vi "SRV_Write_Comm.vi"(8 "error in (no error)":errorcluster, 10 "Command Sent":string, 11 "SRV In":refnum<k5>) -> (0 "error out":errorcluster, 2 "Command Sent dup":string, 3 "SRV Out":refnum<k5>)   [LabVIEW 2014]
doc: "Writes a string to the SRV.\n\n\nWritten for Benilde St. Margaret's School - Tim Jump\nBy Doug Schmertman - Logic PD\nCopyright 2012"
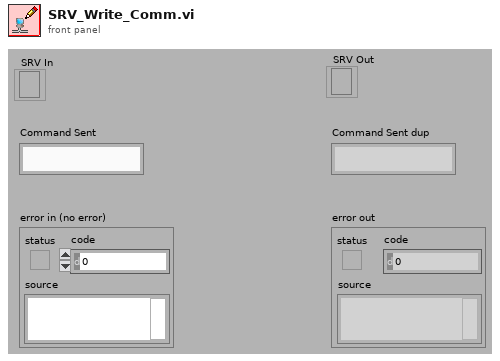
[diagram p1: front panel]
types:
  T1 = typedef "SRV_PM_Packet Mode Style.ctl" = enum16{"Old", "New PM"}
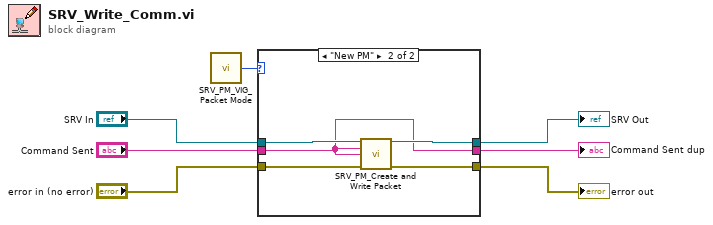
[diagram p0: block diagram]
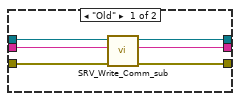
[diagram p2: hidden frame]
diagram:
  n1 = call "SRV_PM_VIG_Packet Mode.vi"() -> ("Packet Mode Style"=w1:T1)  [unwired: 15 in]
  n2 = case shown="\"New PM\"" w1 {
    tunnel: "SRV In" -> [w13 w15]
    tunnel: "error in (no error)" -> [w12 w18]
    tunnel: "Command Sent" -> [w11 w14]
    tunnel: [w10 w14] -> w4
    tunnel: [w9 w16] -> w3
    tunnel: [w8 w17] -> w2
    frame "Old" {
      n3 = call "SRV_Write_Comm_sub.vi"("error in (no error)"=w12, "Command Sent"=w11, "SRV In"=w13) -> ("error out"=w8:errorcluster, "Command Sent dup"=w10:string, "SRV Out"=w9:refnum<k5>)  [unwired: 6 in]
    }
    frame "New PM" {
      n4 = call "SRV_PM_Create and Write Packet.vi"("SRV ref"=w15, "Command Type"=w14, "Data String"=w14, "error in (no error)"=w18) -> ("SRV ref out"=w16:refnum<k5>, "error out"=w17:errorcluster)  [unwired: 10 in]
    }
  }
  "SRV Out" <- w3
  "error out" <- w2
  "Command Sent dup" <- w4
